vi "Get All Formula Parsing VI Variables.vi"() -> (0 "All Variables":string[](array[string]))   [LabVIEW 2020]
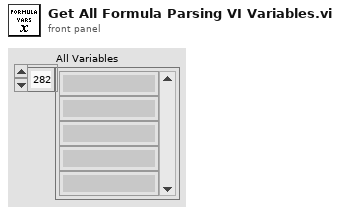
[diagram p1: front panel]
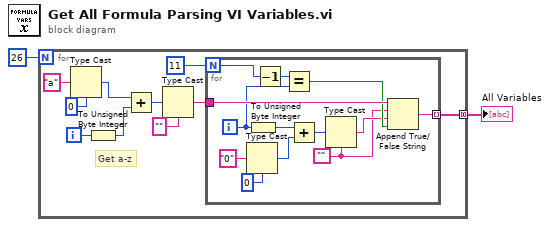
[diagram p0: block diagram]
diagram:
  n1 = for {
    N: 26 -> [_]
    tunnel: [w11] -> w2 mode=concatenating
    i -> [w7]
    # "Get a-z"
    n2 = Type Cast(type=u8 0, x="a") -> (*(type *) &x=w5:u8)
    n3 = To Unsigned Byte Integer(number=w7) -> (unsigned 8bit integer=w4:u8)
    n4 = Add(x=w5, y=w4) -> (x+y=w3:u8)
    n5 = Type Cast(type="", x=w3) -> (*(type *) &x=w6:string)
    n6 = for {
      N: 11 -> [w16]
      tunnel: [w23] -> w11 mode=indexing
      tunnel: w6 -> [w25]
      i -> [w17]
      w14 = "" ("type")
      n7 = Type Cast(type=u8 0, x="0") -> (*(type *) &x=w18:u8)
      n8 = To Unsigned Byte Integer(number=w17) -> (unsigned 8bit integer=w21:u8)
      n9 = Decrement(x=w16) -> (x-1=w13:i32)
      n10 = Equal?(x=w13, y=w17) -> (x = y?=w24:bool)
      n11 = Add(x=w21, y=w18) -> (x+y=w22:u8)
      n12 = Type Cast(type=w14, x=w22) -> (*(type *) &x=w15:string)
      n13 = Append True/False String(1:w24, 2:w15, 3:w14, 4:w25) -> (0:w23:string)
    }
  }
  "All Variables" <- w2
